vi "Day 9 Puzzle 1.vi"(11 "Path":path) -> ()   [LabVIEW 2021]
uses:
  SubVIs/Positions.ctl
  <vilib>/Utility/file.llb/Read Delimited Spreadsheet (string).vi
  <userlib>/_OpenG.lib/array/array.llb/Remove Duplicates from 1D Array (Variant)__ogtk.vi
panel:
  out "Numeric":i32
  out "size(s) 2":i32
  out "Array":T1[](array[typedef])
  out "size(s)":i32
  out "Head Positions":T1[](array[typedef])
  out "Head Position":T1
  out "Tail Position":T1
  out "list of movements":string[][](array[string])
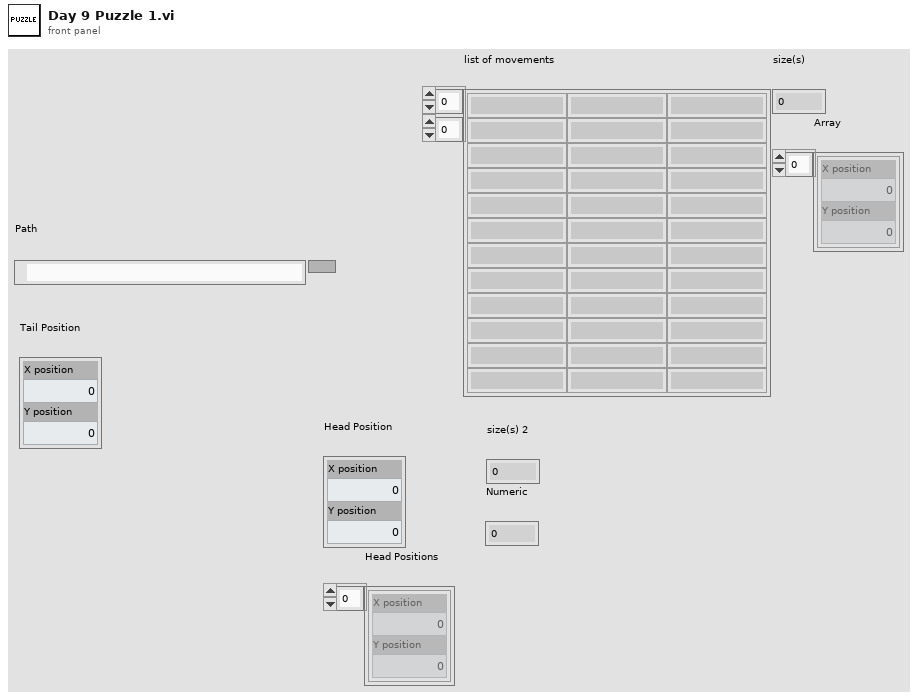
[diagram p1: front panel]
types:
  T1 = typedef "Positions.ctl" = cluster{"X position":i32, "Y position":i32}
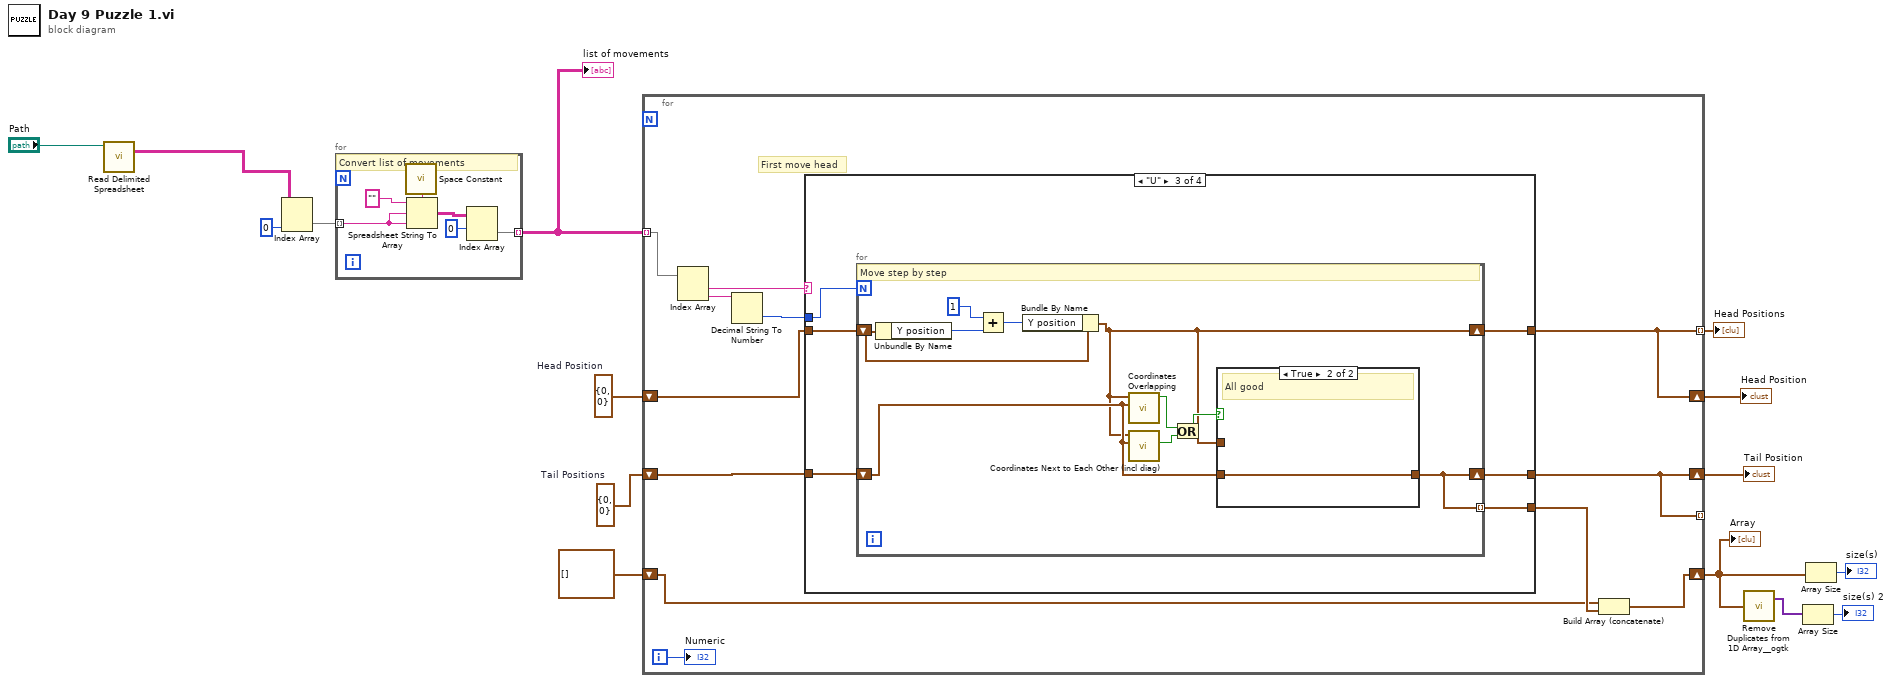
[diagram p0: block diagram]
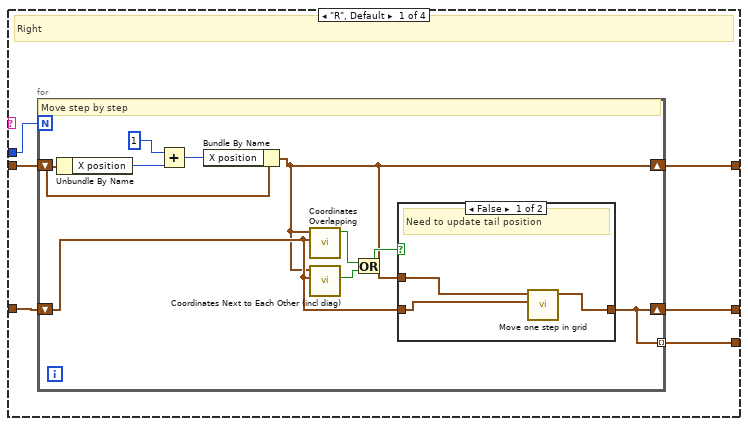
[diagram p2: hidden frame]
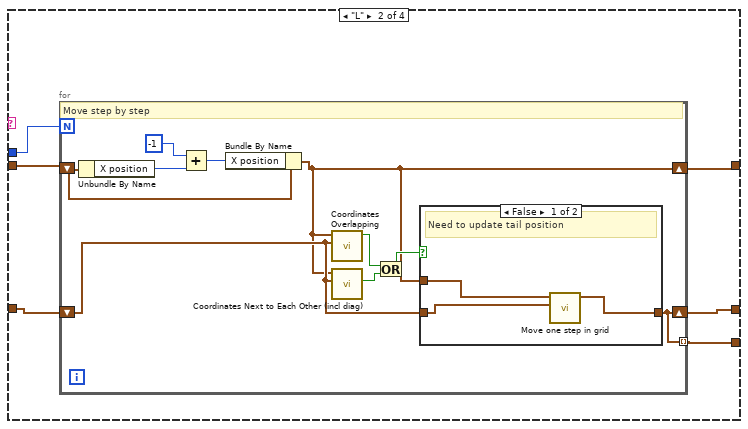
[diagram p4: hidden frame]
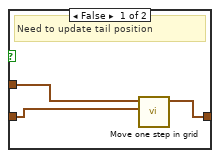
[diagram p6: hidden frame]
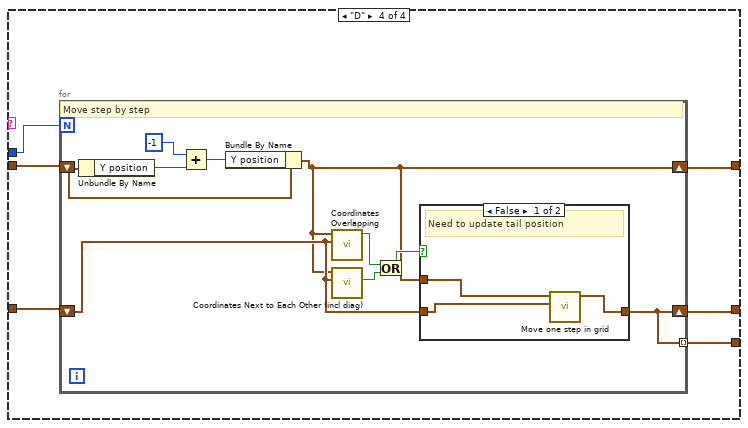
[diagram p7: hidden frame]
diagram:
  w6 = T1 {"X position"=0, "Y position"=0}  # Tail Positions
  w11 = T1 {"X position"=0, "Y position"=0}  # Head Position
  n1 = call-poly <vilib>:"Read Delimited Spreadsheet.vi"("file path (dialog if empty)"="Path") -> ("all rows"=w14:string[][])  [unwired: 9 in, 5 out]
  n2 = Index Array(array=w14, index (col)=0 ("disabled index (col)")) -> (element=w12:string[])  [unwired: 1 in]
  n3 = for {
    tunnel: [w18] -> w1 mode=indexing
    tunnel: w12 -> [w16] mode=indexing
    # "Convert list of movements"
    n4 = call <vilib>:"Space Constant.vi"() -> ("String"=w20:string)
    n5 = Spreadsheet String To Array(delimiter (Tab)=w20, format string="", spreadsheet string=w16, array type (2D Dbl)=w16) -> (array=w17:string[][])
    n6 = Index Array(array=w17, index (row)=0) -> (element=w18:string[])  [unwired: 1 in]
  }
  "list of movements" <- w1
  n7 = for {
    tunnel: w1 -> [w33] mode=indexing
    shift-right: [w27] -> w9
    shift-left: w11 -> [w31]
    shift-right: [w26] -> w10
    shift-left: w6 -> [w28]
    tunnel: [w27] -> w8 mode=indexing
    tunnel: [w26] -> _ mode=indexing
    shift-right: [w23] -> w4
    shift-left: T1[] [] -> [w24]
    i -> [w22]
    # "First move head"
    n8 = Index Array(array=w33) -> (element #1=w32:string, element #2=w30:string)  [unwired: 2 in]
    n9 = Decimal String To Number(string=w30) -> (number=w29:i32)  [unwired: 2 in, 1 out]
    n10 = case shown="\"U\"" w32 {
      tunnel: w31 -> [w39 w59 w79 w99]
      tunnel: w29 -> [w37 w55 w78 w98]
      tunnel: [w38 w57 w77 w97] -> w27
      tunnel: w28 -> [w36 w58 w75 w95]
      tunnel: [w35 w56 w76 w96] -> w26
      tunnel: [w34 w54 w74 w94] -> w25
      frame "R", Default {
        # "Right"
        n11 = for {
          N: w37 -> [_]
          shift-right: [w41] -> w38
          shift-left: w39 -> [w46]
          shift-right: [w40] -> w35
          shift-left: w36 -> [w42]
          tunnel: [w40] -> w34 mode=indexing
          # "Move step by step"
          n12 = Unbundle By Name(w46) -> ("X position"=w49:i32)
          n13 = Add(x=1, y=w49) -> (x+y=w48:i32)
          n14 = Bundle By Name(cluster=w46, "X position"=w48) -> (w41:T1)
          n15 = call "Coordinates Overlapping.vi"("Tail Positions"=w42, "Head Position"=w41) -> ("Checkbox"=w45:bool)  [unwired: 9 in]
          n16 = call "Coordinates Next to Each Other (incl diag).vi"("Tail Positions"=w42, "Head Position"=w41) -> ("Neighbouring"=w44:bool)  [unwired: 8 in, 1 out]
          n17 = Or(x=w45, y=w44) -> (x .or. y?=w43:bool)
          n18 = case shown="False" w43 {
            tunnel: w42 -> [w51 w53]
            tunnel: [w50 w53] -> w40
            tunnel: w41 -> [w52 _]
            frame False {
              # "Need to update tail position"
              n19 = call "Move one step in grid.vi"("Tail Positions"=w51, "Head Position"=w52) -> ("New Tail Position"=w50:T1)  [unwired: 9 in]
            }
            frame True {
              # "All good"
            }
          }
        }
      }
      frame "L" {
        n20 = for {
          N: w55 -> [_]
          shift-right: [w61] -> w57
          shift-left: w59 -> [w66]
          shift-right: [w60] -> w56
          shift-left: w58 -> [w62]
          tunnel: [w60] -> w54 mode=indexing
          # "Move step by step"
          n21 = Unbundle By Name(w66) -> ("X position"=w69:i32)
          n22 = Add(x=-1, y=w69) -> (x+y=w68:i32)
          n23 = Bundle By Name(cluster=w66, "X position"=w68) -> (w61:T1)
          n24 = call "Coordinates Overlapping.vi"("Tail Positions"=w62, "Head Position"=w61) -> ("Checkbox"=w65:bool)  [unwired: 9 in]
          n25 = call "Coordinates Next to Each Other (incl diag).vi"("Tail Positions"=w62, "Head Position"=w61) -> ("Neighbouring"=w64:bool)  [unwired: 8 in, 1 out]
          n26 = Or(x=w65, y=w64) -> (x .or. y?=w63:bool)
          n27 = case shown="False" w63 {
            tunnel: w62 -> [w71 w73]
            tunnel: [w70 w73] -> w60
            tunnel: w61 -> [w72 _]
            frame False {
              # "Need to update tail position"
              n28 = call "Move one step in grid.vi"("Tail Positions"=w71, "Head Position"=w72) -> ("New Tail Position"=w70:T1)  [unwired: 9 in]
            }
            frame True {
              # "All good"
            }
          }
        }
      }
      frame "U" {
        n29 = for {
          N: w78 -> [_]
          shift-right: [w81] -> w77
          shift-left: w79 -> [w86]
          shift-right: [w80] -> w76
          shift-left: w75 -> [w82]
          tunnel: [w80] -> w74 mode=indexing
          # "Move step by step"
          n30 = Unbundle By Name(w86) -> ("Y position"=w89:i32)
          n31 = Add(x=1, y=w89) -> (x+y=w88:i32)
          n32 = Bundle By Name(cluster=w86, "Y position"=w88) -> (w81:T1)
          n33 = call "Coordinates Overlapping.vi"("Tail Positions"=w82, "Head Position"=w81) -> ("Checkbox"=w85:bool)  [unwired: 9 in]
          n34 = call "Coordinates Next to Each Other (incl diag).vi"("Tail Positions"=w82, "Head Position"=w81) -> ("Neighbouring"=w84:bool)  [unwired: 8 in, 1 out]
          n35 = Or(x=w85, y=w84) -> (x .or. y?=w83:bool)
          n36 = case shown="True" w83 {
            tunnel: w82 -> [w91 w93]
            tunnel: [w90 w93] -> w80
            tunnel: w81 -> [w92 _]
            frame False {
              # "Need to update tail position"
              n37 = call "Move one step in grid.vi"("Tail Positions"=w91, "Head Position"=w92) -> ("New Tail Position"=w90:T1)  [unwired: 9 in]
            }
            frame True {
              # "All good"
            }
          }
        }
      }
      frame "D" {
        n38 = for {
          N: w98 -> [_]
          shift-right: [w101] -> w97
          shift-left: w99 -> [w106]
          shift-right: [w100] -> w96
          shift-left: w95 -> [w102]
          tunnel: [w100] -> w94 mode=indexing
          # "Move step by step"
          n39 = Unbundle By Name(w106) -> ("Y position"=w109:i32)
          n40 = Add(x=-1, y=w109) -> (x+y=w108:i32)
          n41 = Bundle By Name(cluster=w106, "Y position"=w108) -> (w101:T1)
          n42 = call "Coordinates Overlapping.vi"("Tail Positions"=w102, "Head Position"=w101) -> ("Checkbox"=w105:bool)  [unwired: 9 in]
          n43 = call "Coordinates Next to Each Other (incl diag).vi"("Tail Positions"=w102, "Head Position"=w101) -> ("Neighbouring"=w104:bool)  [unwired: 8 in, 1 out]
          n44 = Or(x=w105, y=w104) -> (x .or. y?=w103:bool)
          n45 = case shown="False" w103 {
            tunnel: w102 -> [w111 w113]
            tunnel: [w110 w113] -> w100
            tunnel: w101 -> [w112 _]
            frame False {
              # "Need to update tail position"
              n46 = call "Move one step in grid.vi"("Tail Positions"=w111, "Head Position"=w112) -> ("New Tail Position"=w110:T1)  [unwired: 9 in]
            }
            frame True {
              # "All good"
            }
          }
        }
      }
    }
    n47 = Build Array (concatenate)(w24, w25) -> (w23:T1[])
    "Numeric" <- w22
  }
  "Tail Position" <- w10
  "Head Position" <- w9
  "Head Positions" <- w8
  "Array" <- w4
  n48 = call-poly <userlib>:"Remove Duplicates from 1D Array__ogtk.vi"("Input Array"=w4) -> ("Output Array"=w2:variant[])  [unwired: 1 out]
  n49 = Array Size(array=w2) -> (size(s)=→"size(s) 2":i32)
  n50 = Array Size(array=w4) -> (size(s)=→"size(s)":i32)
